vi "TTM 3He Press to Temp.vi"(1 "3He Vapor pressure in mmhg  between  0.02 and 200.":dbl format="%.4f") -> (0 "corresponding temp K":dbl format="%.3f")   [LabVIEW 2009]
doc: "This VI use a spline fitting routine to convert helium vapor pressures to temperature. Select wither He3 or He4, type in the pressure and the temperature is returned."
uses:
  <vilib>/Analysis/NI_AALPro.lvlib
panel:
  in  "interpolant he3":dbl[](array[numeric])=[1013.2888925508655, -304.57778510173074, 41.088909029758995, -29.277851017304894, -1.9775049605391548, -4.812129140538857, -0.9553890705988911, -0.7263145770655806, -0.3993526211387837, -0.2562749383792669, -0.19554762534417008, -0.1615345602439872, -0.11831413367997518, -0.08520890503603276, -0.0808502461759675, -0.03611762817046551, -0.024279241142169602, -0.015565407260855684, -0.011859129814407482, -0.00899807348151445, -0.007348576259536633, -0.004655234480632103, -0.0034304858179350474, -0.0032228222476273273, -0.0016782251915563261, -0.0020642769861467128, -0.001464666863857566, -0.001023860915353568, -0.0008898894747284509, -0.000666581185732383, -0.000493785782342237, -0.0005082756848986551, -0.00028731376934682055, -0.00023846923771406707, -0.00017480927979696836, -0.00014229364309799382, -0.00012001614781106781, -9.764176565776223e-05, -7.306662912117246e-05, -5.4091717857552326e-05, -4.656649944860788e-05, -3.564228434802573e-05, -3.286436315927807e-05, -2.4900263014867483e-05, -2.3534584781261462e-05, -1.8961397860071477e-05, -2.0619823778466065e-05, -1.2559307026051709e-05, -1.9142948117330513e-05, 5.131099495369689e-06, -8.538144986413898e-05, 0.00027039469996118024, -0.0010621973499805879] format="%.2f"
  in  "pressure array":dbl[](array[numeric])=[0.01, 0.02, 0.04, 0.06, 0.08, 0.1, 0.2, 0.3, 0.4, 0.5, 0.6, 0.7, 0.8, 0.9, 1.0, 1.5, 2.0, 2.5, 3.0, 3.5, 4.0, 5.0, 6.0, 7.0, 8.0, 9.0, 10.0, 12.0, 14.0, 16.0, 18.0, 20.0, 25.0, 30.0, 35.0, 40.0, 45.0, 50.0, 60.0, 70.0, 80.0, 90.0, 100.0, 110.0, 120.0, 130.0, 140.0, 150.0, 160.0, 170.0, 180.0, 190.0, 200.0] format="%.4f"
  in  "He3  T array":dbl[](array[numeric])=[0.3557, 0.3844, 0.4174, 0.4391, 0.4556, 0.4693, 0.5163, 0.5477, 0.572, 0.592, 0.6093, 0.6246, 0.6383, 0.6508, 0.6624, 0.7101, 0.7474, 0.7785, 0.8055, 0.8295, 0.8512, 0.8894, 0.9227, 0.9524, 0.9791, 1.0038, 1.0266, 1.0679, 1.1049, 1.1384, 1.1692, 1.1979, 1.2617, 1.3176, 1.3676, 1.4131, 1.455, 1.4939, 1.5646, 1.6279, 1.6856, 1.7387, 1.7881, 1.8343, 1.8779, 1.9192, 1.9585, 1.9959, 2.0318, 2.0663, 2.0994, 2.1314, 2.1623] format="%.4f"
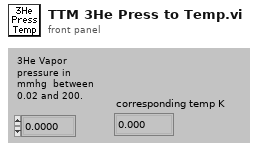
[diagram p1: front panel]
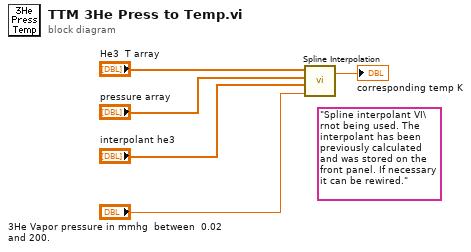
[diagram p0: block diagram]
diagram:
  (unwired) "Spline interpolant VI\rnot being used. The interpolant has been previously calculated and was stored on the front panel. If necessary it can be rewired."
  n1 = call <vilib>:"Spline Interpolation.vi"("x value"="3He Vapor pressure in mmhg  between  0.02 and 200.", "Interpolant"="interpolant he3", "X"="pressure array", "Y"="He3  T array") -> ("interpolation value"=→"corresponding temp K":dbl)  [unwired: 1 out]
